vi "RP Read RX FIFO Fast TCP.vi"(6 "Samples per read":i32=1024, 7 "bytes per sample":i32=12, 8 "Error In":errorcluster, 11 "connection ID":refnum<k5>) -> (0 "Error Out":errorcluster, 2 "FIFO out":i32[](array[numeric]), 3 "connection ID out":refnum<k5>)   [LabVIEW 2019]
uses:
  RP Command.ctl
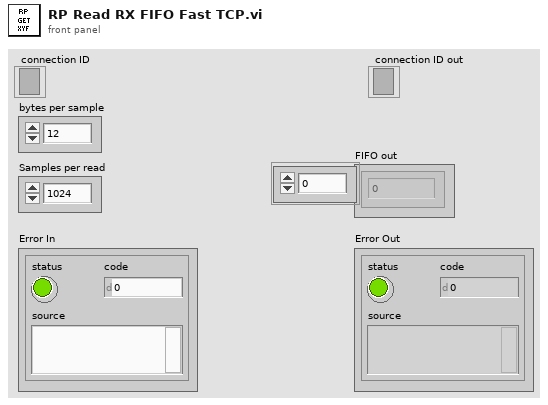
[diagram p1: front panel]
types:
  T1 = typedef "RP Command.ctl" = enum16{"Reset", "Read IDN", "Stop server", "Get status", "Get temperature", "Connect client", "Arm", "Software trigger", "Get whole buffer", "Get chunk", "System call", "Get config", "Set config", "Recieve data", "Recieve Calibartion", "Transmit data"}
  T2 = enum16{"big-endian, network order", "native, host order", "little-endian"}
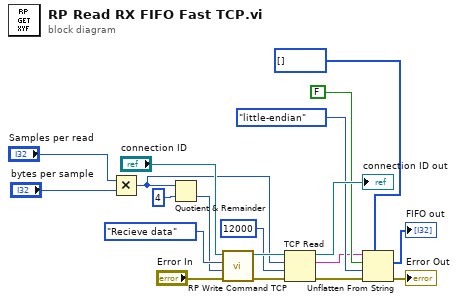
[diagram p0: block diagram]
diagram:
  n1 = Multiply(x="Samples per read", y="bytes per sample") -> (x*y=w2:i32)
  n2 = Quotient & Remainder(x=w2, y=4) -> (floor(x/y)=w1:i32)  [unwired: 1 out]
  n3 = call "RP Write Command TCP.vi"("Error In"="Error In", "Command payload"=w1, "Command number"=RP_Command."Recieve data", "connection ID"="connection ID") -> ("Error Out"=w18:errorcluster, "connection ID out"=w19:refnum<k5>)  [unwired: 5 in, 1 out]
  n4 = TCP Read(connection ID=w19, bytes to read=w2, error in (no error)=w18, 9:12000 ("timeout ms (25000)")) -> (connection ID out=→"connection ID out":refnum<k5>, data out=w10:string, error out=w9:errorcluster)  [unwired: 1 in]
  n5 = Unflatten From String(type=i32[] [], binary string=w10, data includes array or string size? (T)=FALSE, byte order (0:big-endian, network order)=T2."little-endian", error in (no error)=w9) -> (value=→"FIFO out":i32[], error out=→"Error Out":errorcluster)  [unwired: 1 out]
